vi "Control.vi"(11 "?":T1) -> (2 "Right Joy Stick":dbl, 3 "Left Joy Stick":dbl)   [LabVIEW 2014]
uses:
  SRE Enum.ctl
  <vilib>/Rock Robotics/WPI/Joystick/WPI_JoystickDeviceEnum.ctl
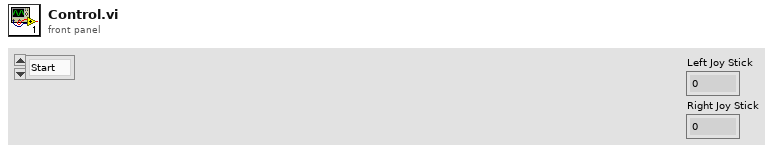
[diagram p1: front panel]
types:
  T1 = typedef "SRE Enum.ctl" = enum16{"Start", "Run", "End"}
  T2 = typedef "WPI_JoystickDeviceEnum.ctl" = enum16{"USB 0", "USB 1", "USB 2", "USB 3", "USB 4", "USB 5"}
  T3 = typedef "WPI_JoystickDevRef.ctl" = cluster{"Device":T2}
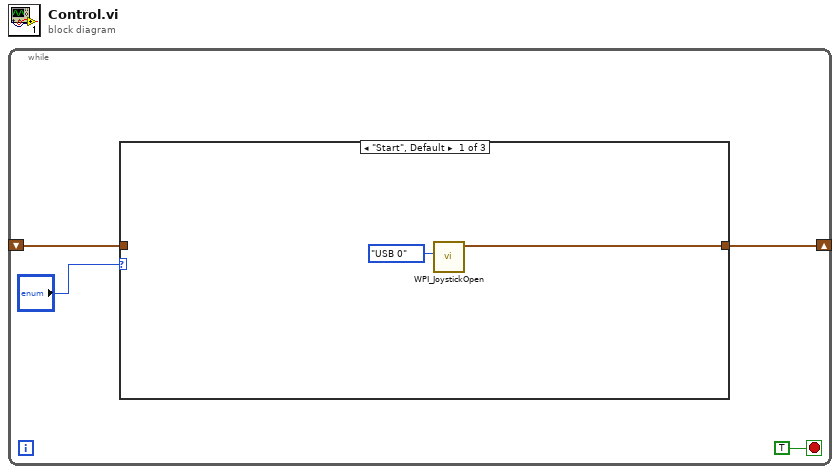
[diagram p0: block diagram]
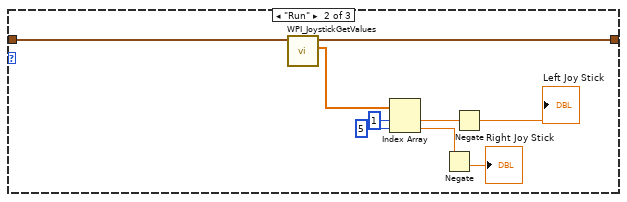
[diagram p2: hidden frame]
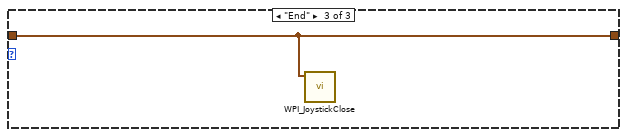
[diagram p3: hidden frame]
diagram:
  n1 = while {
    shift-right: [w3] -> _
    shift-left: _ -> [w2]
    stop <- TRUE stop-if-true
    n2 = case shown="\"Start\", Default" "?" {
      tunnel: [w6 w14 w16] -> w3
      tunnel: w2 -> [_ w15 w16]
      frame "Start", Default {
        n3 = call <vilib>:"WPI_JoystickOpen.vi"("JoystickDevice"=WPI_JoystickDeviceEnum."USB 0") -> ("JoystickDevRef"=w6:T3)  [unwired: 10 in]
      }
      frame "Run" {
        n4 = call <vilib>:"WPI_JoystickGetValues.vi"("JoystickDevRef"=w15) -> ("Axes"=w13:dbl[], "JoystickDevRef"=w14:T3)  [unwired: 6 in, 3 out]
        n5 = Index Array(array=w13, index #1=1 ("index"), index #2=5 ("index")) -> (element #1=w10:dbl, element #2=w9:dbl)
        n6 = Negate(x=w9) -> (-x=→"Right Joy Stick":dbl)
        n7 = Negate(x=w10) -> (-x=→"Left Joy Stick":dbl)
      }
      frame "End" {
        n8 = call <vilib>:"WPI_JoystickClose.vi"("JoystickDevRef"=w16) -> ()  [unwired: 11 in]
      }
    }
  }
